vi "ResetCAN.vi"(8 "error in (no error)":errorcluster caption="错误输入（无错误）", 9 "CANInd":u32, 10 "DeciceInd":u32, 11 "DeviceType":u32) -> (0 "error out":errorcluster caption="错误输出", 3 "Valid":bool)   [LabVIEW 2011]
uses:
  data/ControlCAN.dll
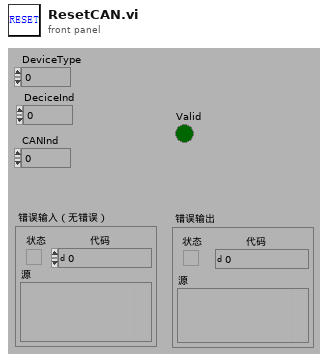
[diagram p1: front panel]
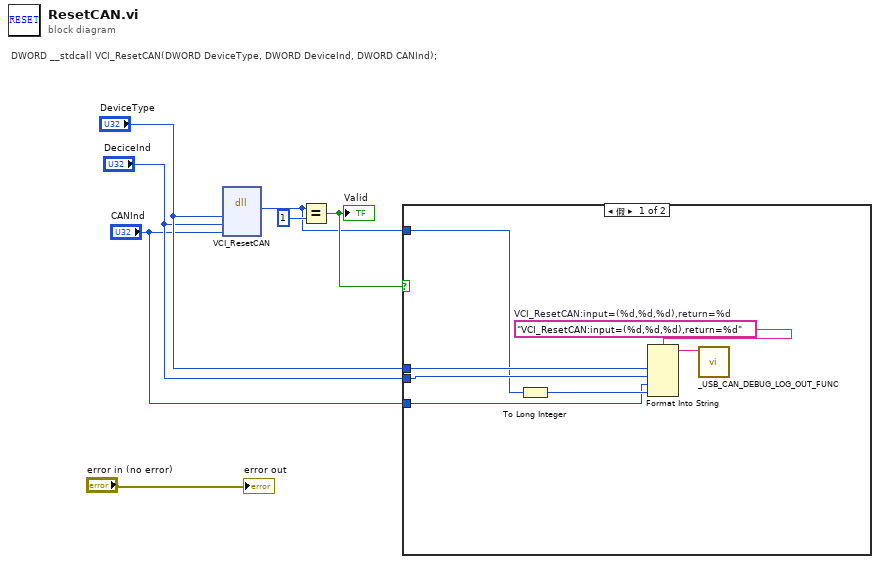
[diagram p0: block diagram]
diagram:
  # "DWORD __stdcall VCI_ResetCAN(DWORD DeviceType, DWORD DeviceInd, DWORD CANInd);"
  n1 = dll-call lib="PTH1Mabs ZHost_E工作TnewcodeUSB CAN Tool1.97dataControlCAN.dll" fn="VCI_ResetCAN"("DeviceType"="DeviceType", "DeciceInd"="DeciceInd", "CANInd"="CANInd") -> ("返回类型"=w4:u32)  [unwired: 6 in, 2 out]
  n2 = Equal?(x=w4, y=u32 1) -> (x = y?=w5:bool)
  "Valid" <- w5
  n3 = case shown="假" w5 {
    tunnel: "DeviceType" -> [w13 _]
    tunnel: "DeciceInd" -> [w12 _]
    tunnel: w4 -> [w11 _]
    tunnel: "CANInd" -> [w8 _]
    frame False {
      w10 = "VCI_ResetCAN:input=(%d,%d,%d),return=%d"  # VCI_ResetCAN:input=(%d,%d,%d),return=%d
      n4 = To Long Integer(number=w11) -> (32bit integer=w9:i32)
      n5 = Format Into String(format string=w10, w13, w12, w8, w9) -> (resulting string=w14:string)  [unwired: 2 in, 1 out]
      n6 = call "_USB_CAN_DEBUG_LOG_OUT_FUNC.vi"("Info"=w14) -> ()  [unwired: 11 in]
    }
    frame True {
    }
  }
  "error out" <- "error in (no error)"
